vi "config_in_line_OSC.vi"(8 "error in (no error)":errorcluster, 11 "OSC 2":refnum<visa-resource-name>) -> (0 "error out":errorcluster, 3 "VISA resource name out":refnum<visa-resource-name>)   [LabVIEW 2011]
uses:
  SubVIs/scale.ctl
  SubVIs/sampling_rate.ctl
  <instrlib>/Tektronix 7000 Series/Public/Configure/Configure Trigger (Edge).vi
  <instrlib>/Tektronix 7000 Series/Tektronix 7000 Series.lvlib
panel:
  in  "configure":bool
  out "resolution (Hz)":ext format="%#_6p"
  out "sampling interval (s)":ext format="%#_6p"
  out "waveform length (s)":ext format="%#_6p"
  in  "horizontal scale (t/div)":T1=4e-7 items=["400ns/div", "1µs/div", "2µs/div", "4µs/div", "10µs/div", "20µs/div"]
  in  "sampling rate (Hz)":T2=20000000000.0 items=["20 GHz (50ps/sample)", "10 GHz (100ps/sample)", "5.0 GHz (200ps/sample)", "2.5 GHz (400ps/sample)", "1.25 GHz (0.8ns/sample)", "0.5 GHz (2ns/sample)"]
  out "sample points":i32
  in  "Trigger Level":dbl=1.0 format="%.1f"
  in  "CH2 Vertical Offset":dbl=6.0 format="%.1g"
  in  "CH2 Vertical Range":dbl=7.0 format="%.1g"
  in  "CH2 Input Impedance":enum16{"1M", "50"}(ring)=enum."50"
  in  "CH1 Input Impedance":enum16{"1M", "50"}(ring)
  in  "CH1 Vertical Range":dbl=10.0
  in  "RESET?":bool
  in  "STOP":bool
  # "Configure Oscilloscope"
  # "CH2 - Trigger Input Channel"
  # "CH1 - Microwave Input Channel"
  # "Resolution and Record Length"
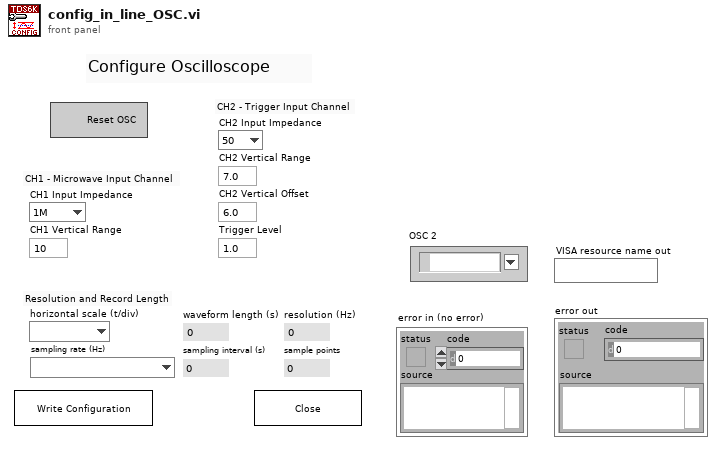
[diagram p1: front panel]
types:
  T1 = typedef "scale.ctl" = ext
  T2 = typedef "sampling_rate.ctl" = ext
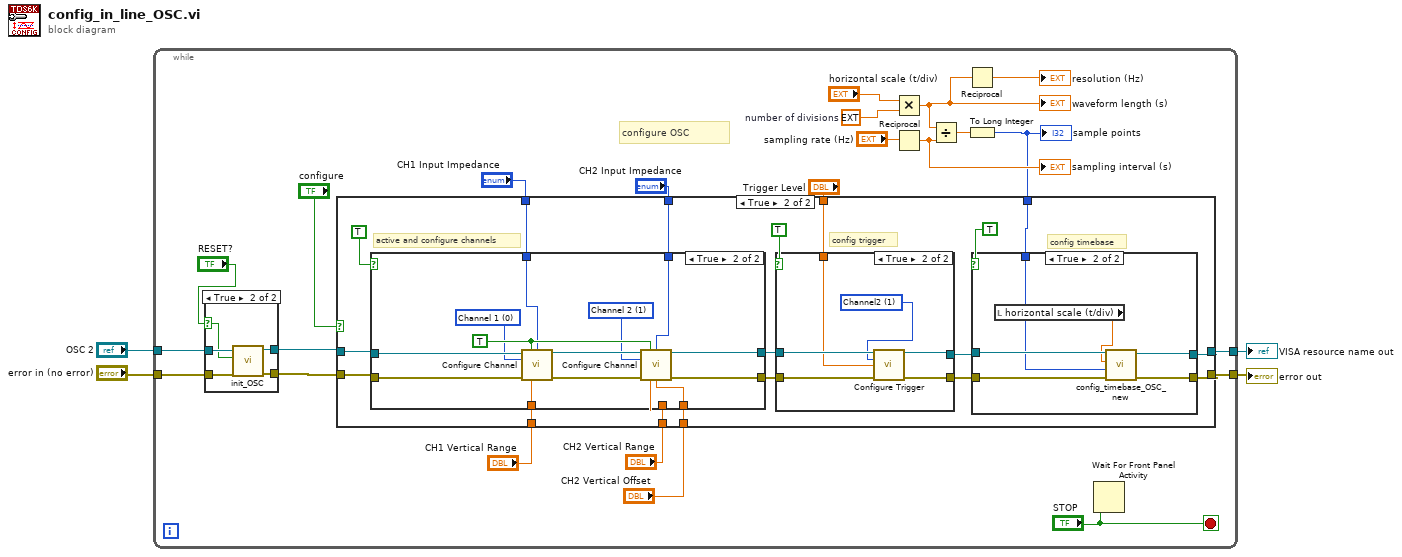
[diagram p0: block diagram]
diagram:
  n1 = while {
    tunnel: "OSC 2" -> [w9]
    tunnel: "error in (no error)" -> [w8]
    tunnel: [w23] -> w2
    tunnel: [w22] -> w1
    stop <- "STOP" stop-if-true
    w27 = ext 10.0  # number of divisions
    # "configure OSC"
    n2 = case shown="True" "RESET?" {
      selector: "RESET?" -> [_ w30]
      tunnel: w9 -> [w29 w34]
      tunnel: w8 -> [w28 w33]
      tunnel: [w28 w32] -> w7
      tunnel: [w29 w31] -> w6
      frame False {
      }
      frame True {
        n3 = call "init_OSC.vi"("error in (no error)"=w33, "reset (f)"=w30, "VISA resource name"=w34) -> ("error out"=w32:errorcluster, "VISA resource name out"=w31:refnum<visa-resource-name>)  [unwired: 7 in]
      }
    }
    n4 = Multiply(x="horizontal scale (t/div)", y=w27) -> (x*y=w12:T1)
    "waveform length (s)" <- w12
    n5 = Reciprocal(x="sampling rate (Hz)") -> (1/x=w16:T2)
    "sampling interval (s)" <- w16
    n6 = Divide(x=w12, y=w16) -> (x/y=w15:T1)
    n7 = Reciprocal(x=w12) -> (1/x=→"resolution (Hz)":T1)
    n8 = To Long Integer(number=w15) -> (32bit integer=w14:i32)
    "sample points" <- w14
    n9 = case shown="True" "configure" {
      tunnel: w6 -> [w36 w37]
      tunnel: w7 -> [w35 w38]
      tunnel: [w36 w48] -> w23
      tunnel: [w35 w47] -> w22
      tunnel: "CH1 Vertical Range" -> [_ w45]
      tunnel: "CH2 Vertical Offset" -> [_ w44]
      tunnel: "CH2 Vertical Range" -> [_ w43]
      tunnel: "CH2 Input Impedance" -> [_ w42]
      tunnel: "CH1 Input Impedance" -> [_ w41]
      tunnel: "Trigger Level" -> [_ w40]
      tunnel: w14 -> [_ w39]
      frame False {
      }
      frame True {
        # "config timebase"
        # "config trigger"
        # "active and configure channels"
        n10 = case shown="True" TRUE ("channel") {
          tunnel: w37 -> [w72 w84]
          tunnel: w38 -> [w71 w83]
          tunnel: [w72 w82] -> w52
          tunnel: [w71 w81] -> w51
          tunnel: w45 -> [_ w79]
          tunnel: w44 -> [_ w78]
          tunnel: w43 -> [_ w77]
          tunnel: w42 -> [_ w76]
          tunnel: w41 -> [_ w74]
          frame False {
          }
          frame True {
            w75 = u16 1 items=["Channel 1", "Channel 2", "Channel 3", "Channel 4", "Math 1", "Math 2", "Math 3", "Math 4", "Reference 1", "Reference 2", "Reference 3", "Reference 4"] ("Channel (0: Channel 1)")
            w80 = TRUE ("Enable Channel (T: Enable)")
            w73 = u16 0 items=["Channel 1", "Channel 2", "Channel 3", "Channel 4", "Math 1", "Math 2", "Math 3", "Math 4", "Reference 1", "Reference 2", "Reference 3", "Reference 4"] ("Channel (0: Channel 1)")
            n11 = call <instrlib>:"Configure Channel.vi"("VISA resource name"=w84, "Enable Channel (T: Enable)"=w80, "Input Impedance (0: 1M ohm)"=w74, "Channel (0: Channel 1)"=w73, "error in (no error)"=w83, "Vertical Range (10.0 V)"=w79) -> ("VISA resource name out"=w85:refnum<visa-resource-name>, "error out"=w86:errorcluster)  [unwired: 8 in]
            n12 = call <instrlib>:"Configure Channel.vi"("VISA resource name"=w85, "Enable Channel (T: Enable)"=w80, "Input Impedance (0: 1M ohm)"=w76, "Channel (0: Channel 1)"=w75, "error in (no error)"=w86, "Vertical Range (10.0 V)"=w77, "Vertical Offset (0.0 V)"=w78) -> ("VISA resource name out"=w82:refnum<visa-resource-name>, "error out"=w81:errorcluster)  [unwired: 7 in]
          }
        }
        n13 = case shown="True" TRUE ("trigger") {
          tunnel: w52 -> [w64 w70]
          tunnel: w51 -> [w63 w69]
          tunnel: [w64 w68] -> w50
          tunnel: [w63 w67] -> w49
          tunnel: w40 -> [_ w66]
          frame False {
          }
          frame True {
            w65 = u16 1 items=["Channel1"=0, "Channel2"=1, "Channel3"=2, "Channel4"=3, "Aux"=12, "Line"=13, "Digital Channel0"=14, "Digital Channel1"=15, "Digital Channel2"=16, "Digital Channel3"=17, "Digital Channel4"=18, "Digital Chennel5"=19, "Digital Channel6"=20, "Digital Channel7"=21, "Digital Channel8"=22, "Digital Channel9"=23, "Digital Channel10"=24, "Digital Channel11"=25, "Digital Channel12"=26, "Digital Channel13"=27, "Digital Channel14"=28, "Digital Channel15"=29] ("Trigger Channel")
            n14 = call-poly <instrlib>:"Configure Trigger.vi"("VISA resource name"=w70, "Source (0:Channel1)"=w65, "Trigger Level (0.0V)"=w66, "error in (no error)"=w69) -> ("VISA resource name out"=w68:refnum<visa-resource-name>, "error out"=w67:errorcluster)  [unwired: 10 in]
          }
        }
        n15 = case shown="True" TRUE ("timebase") {
          tunnel: w50 -> [w56 w62]
          tunnel: w49 -> [w55 w61]
          tunnel: [w56 w59] -> w48
          tunnel: [w55 w60] -> w47
          tunnel: w39 -> [_ w57]
          frame False {
          }
          frame True {
            n16 = local read "horizontal scale (t/div)"() -> (w58:T1)
            n17 = call "config_timebase_OSC_new.vi"("error in (no error)"=w61, "resolution"=w57, "hor scale"=w58, "VISA resource name"=w62) -> ("error out"=w60:errorcluster, "VISA resource name out"=w59:refnum<visa-resource-name>)  [unwired: 5 in, 1 out]
          }
        }
      }
    }
    n18 = Wait For Front Panel Activity(3:"STOP") -> ()  [unwired: 2 in, 1 out]
  }
  "VISA resource name out" <- w2
  "error out" <- w1
